vi "IR_Vibration_sensor_output_digital.vi"() -> ()   [LabVIEW 2022 SP3]
uses:
  <vilib>/DAQmx/read.llb/DAQmx Read (Analog DBL 1Chan 1Samp).vi
  <vilib>/DAQmx/read.llb/DAQmx Read (Digital Bool 1Line 1Point).vi
  <vilib>/DAQmx/write.llb/DAQmx Write (Digital Bool 1Line 1Point).vi
  <vilib>/DAQmx/create/channels.llb/DAQmx Create Channel (DO-Digital Output).vi
  <vilib>/DAQmx/create/channels.llb/DAQmx Create Channel (DI-Digital Input).vi
  <vilib>/DAQmx/create/channels.llb/DAQmx Create Channel (AI-Voltage-Basic).vi
  <vilib>/DAQmx/miscellaneous.llb/DAQmx Fill In Error Info.vi
panel:
  out "Waveform Chart":dbl(graph)
  out "Numeric":dbl
  out "Boolean":bool
  in  "stop":bool
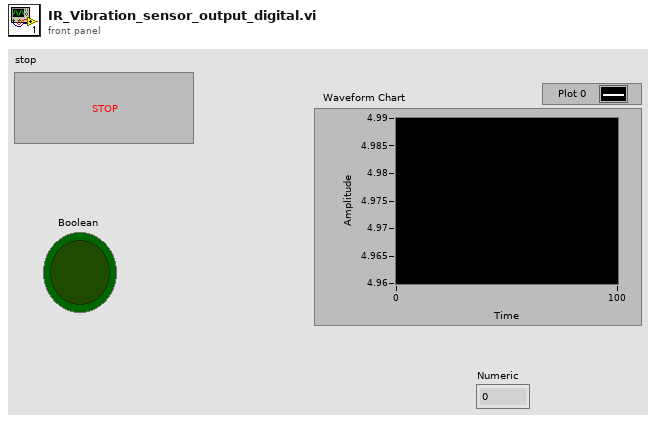
[diagram p1: front panel]
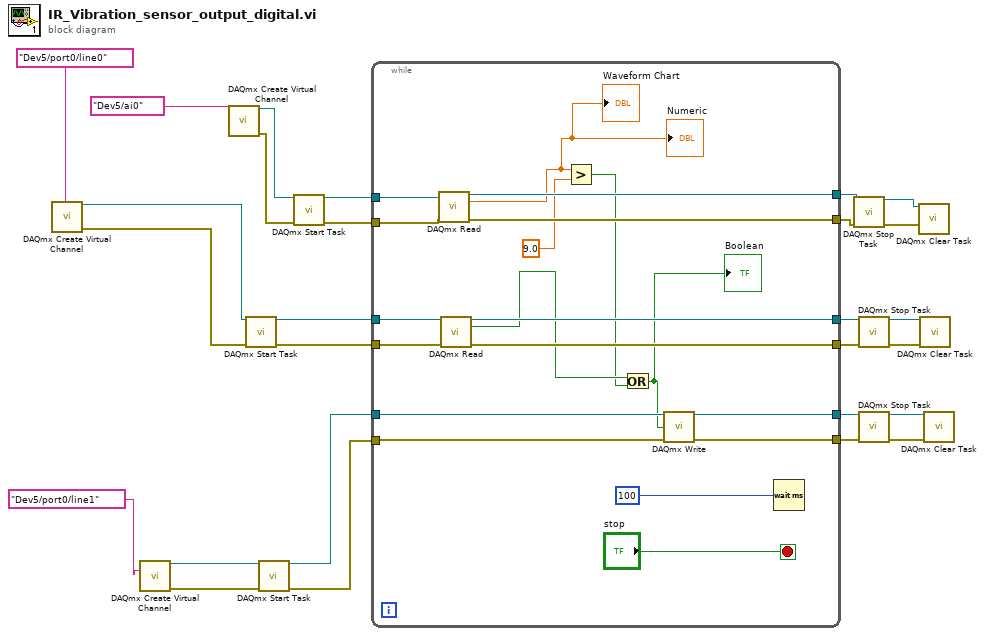
[diagram p0: block diagram]
diagram:
  n1 = call-poly <vilib>:"DAQmx Create Virtual Channel.vi"("lines"=tag "Dev5/port0/line0") -> ("task out"=w12:refnum<k21>, "error out"=w11:errorcluster)  [unwired: 13 in]
  n2 = call-poly <vilib>:"DAQmx Create Virtual Channel.vi"("lines"=tag "Dev5/port0/line1") -> ("task out"=w23:refnum<k21>, "error out"=w18:errorcluster)  [unwired: 13 in]
  n3 = call-poly <vilib>:"DAQmx Create Virtual Channel.vi"("physical channels"=tag "Dev5/ai0") -> ("task out"=w9:refnum<k21>, "error out"=w8:errorcluster)  [unwired: 13 in]
  n4 = call <vilib>:"DAQmx Start Task.vi"("task/channels in"=w12, "error in"=w11) -> ("task out"=w27:refnum<k21>, "error out"=w21:errorcluster)  [unwired: 12 in]
  n5 = call <vilib>:"DAQmx Start Task.vi"("task/channels in"=w23, "error in"=w18) -> ("task out"=w22:refnum<k21>, "error out"=w17:errorcluster)  [unwired: 12 in]
  n6 = call <vilib>:"DAQmx Start Task.vi"("task/channels in"=w9, "error in"=w8) -> ("task out"=w7:refnum<k21>, "error out"=w6:errorcluster)  [unwired: 12 in]
  n7 = while {
    tunnel: w27 -> [w44]
    tunnel: [w43] -> w26
    tunnel: w22 -> [w42]
    tunnel: [w41] -> w14
    tunnel: w21 -> [w40]
    tunnel: [w39] -> w20
    tunnel: w17 -> [w38]
    tunnel: [w37] -> w13
    tunnel: w7 -> [w34]
    tunnel: w6 -> [w33]
    tunnel: [w32] -> w5
    tunnel: [w31] -> w3
    stop <- "stop" stop-if-true
    n8 = call-poly <vilib>:"DAQmx Read.vi"("task/channels in"=w34, "error in"=w33) -> ("task out"=w32:refnum<k21>, "data"=w28:dbl, "error out"=w31:errorcluster)  [unwired: 11 in]
    "Numeric" <- w28
    "Waveform Chart" <- w28
    n9 = call-poly <vilib>:"DAQmx Read.vi"("task/channels in"=w44, "error in"=w40) -> ("task out"=w43:refnum<k21>, "data"=w36:bool, "error out"=w39:errorcluster)  [unwired: 11 in]
    n10 = Greater?(x=w28, y=9.0) -> (0:w29:bool)
    n11 = Or(x=w36, y=w29) -> (x .or. y?=w35:bool)
    "Boolean" <- w35
    n12 = call-poly <vilib>:"DAQmx Write.vi"("task/channels in"=w42, "data"=w35, "error in"=w38) -> ("task out"=w41:refnum<k21>, "error out"=w37:errorcluster)  [unwired: 10 in, 1 out]
    n13 = Wait (ms)(milliseconds to wait=u32 100) -> ()  [unwired: 1 out]
  }
  n14 = call <vilib>:"DAQmx Stop Task.vi"("task/channels in"=w5, "error in"=w3) -> ("task out"=w4:refnum<k21>, "error out"=w2:errorcluster)  [unwired: 12 in]
  n15 = call <vilib>:"DAQmx Stop Task.vi"("task/channels in"=w26, "error in"=w20) -> ("task out"=w25:refnum<k21>, "error out"=w19:errorcluster)  [unwired: 12 in]
  n16 = call <vilib>:"DAQmx Stop Task.vi"("task/channels in"=w14, "error in"=w13) -> ("task out"=w16:refnum<k21>, "error out"=w15:errorcluster)  [unwired: 12 in]
  n17 = call <vilib>:"DAQmx Clear Task.vi"("task in"=w4, "error in"=w2) -> ()  [unwired: 13 in, 1 out]
  n18 = call <vilib>:"DAQmx Clear Task.vi"("task in"=w25, "error in"=w19) -> ()  [unwired: 13 in, 1 out]
  n19 = call <vilib>:"DAQmx Clear Task.vi"("task in"=w16, "error in"=w15) -> ()  [unwired: 13 in, 1 out]
